vi "Volume ROI entry window.vi"(6 "# of planes":i32, 7 "Do not initialise selector values":bool, 8 "ZplaneIndex (zero based)":i32, 10 "Zoom (in)":dbl=1.0 min=1.0 max=10.0 step=0.10000000149011612, 11 "Coordinates":i32[](array[numeric])) -> (1 "Zoom (out)":dbl=1.0 min=1.0 max=10.0 step=0.10000000149011612, 3 "ROIs Info []":T1[](array[typedef]) {"Zoom" min=1.0 max=10.0 step=0.10000000149011612}, 4 "Cancelled":bool)   [LabVIEW 2013]
uses:
  Typedefs/ROI spec.ctl
  Typedefs/ROI ID Enum.ctl
  ROI Entry screen/Typedefs/Volume entry ctrl refs cluster.ctl
  <vilib>/Utility/miscctls.llb/LVPointTypeDef.ctl
  ROI Entry screen/Globals/gl_Volume Entry UI globals.vi
  ROI Entry screen/Globals/gl_ROI Entry UI globals.vi
panel:
  in  "Z-step (planes)":i32=1 min=1 max=17 step=1
  in  "Dual Rectangle":bool
  in  "Zoom":dbl=1.0 min=0.001 max=10.0 step=0.10000000149011612
  in  "Cancel":bool
  in  "Proceed":bool
  in  "Z-plane 2":u16(ring) caption="Z-plane" items=["Z-plane 1", "Z-plane 2", "Z-plane 3", "Z-plane 4", "Z-plane 5", "Z-plane 6", "Z-plane 7", "Z-plane 8", "Z-plane 9", "Z-plane 10", "Z-plane 11", "Z-plane 12", "Z-plane 13", "Z-plane 14", "Z-plane 15", "Z-plane 16", "Z-plane 17", "Z-plane 18", "Z-plane 19", "Z-plane 20", "Z-plane 21", "Z-plane 22", "Z-plane 23", "Z-plane 24", "Z-plane 25", "Z-plane 26", "Z-plane 27", "Z-plane 28", "Z-plane 29", "Z-plane 30", "Z-plane 31", "Z-plane 32", "Z-plane 33", "Z-plane 34", "Z-plane 35", "Z-plane 36", "Z-plane 37", "Z-plane 38", "Z-plane 39", "Z-plane 40", "Z-plane 41", "Z-plane 42", "Z-plane 43", "Z-plane 44", "Z-plane 45", "Z-plane 46", "Z-plane 47", "Z-plane 48", "Z-plane 49", "Z-plane 50", "Z-plane 51"]
  in  "Z-plane 1":u16(ring) caption="Z-plane" items=["Z-plane 1", "Z-plane 2", "Z-plane 3", "Z-plane 4", "Z-plane 5", "Z-plane 6", "Z-plane 7", "Z-plane 8", "Z-plane 9", "Z-plane 10", "Z-plane 11", "Z-plane 12", "Z-plane 13", "Z-plane 14", "Z-plane 15", "Z-plane 16", "Z-plane 17", "Z-plane 18", "Z-plane 19", "Z-plane 20", "Z-plane 21", "Z-plane 22", "Z-plane 23", "Z-plane 24", "Z-plane 25", "Z-plane 26", "Z-plane 27", "Z-plane 28", "Z-plane 29", "Z-plane 30", "Z-plane 31", "Z-plane 32", "Z-plane 33", "Z-plane 34", "Z-plane 35", "Z-plane 36", "Z-plane 37", "Z-plane 38", "Z-plane 39", "Z-plane 40", "Z-plane 41", "Z-plane 42", "Z-plane 43", "Z-plane 44", "Z-plane 45", "Z-plane 46", "Z-plane 47", "Z-plane 48", "Z-plane 49", "Z-plane 50", "Z-plane 51"]
  in  "Volume":bool
  # "To specify a volume from the drawn rectangle, tick the Volume box and select the z-planes between which the volume should be generated.\n \nTo draw two rectangles at precisely the same XY position but on different z-levels, tick the \"Dual Rectangle\" box."
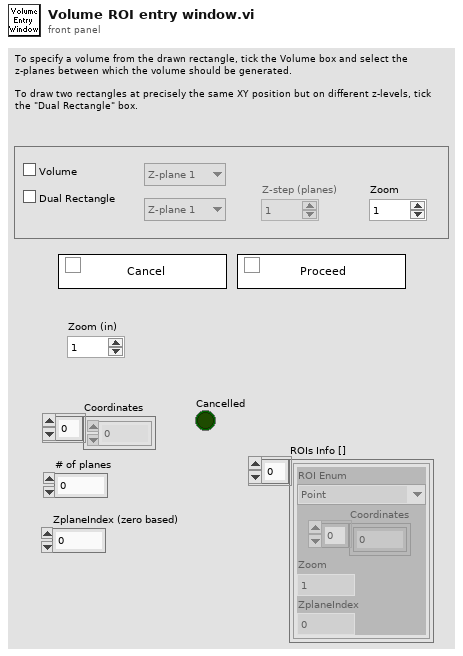
[diagram p1: front panel]
types:
  T1 = typedef "ROI spec.ctl" = cluster{"Coordinates":i32[], "Zoom":dbl, "ROI Enum":T2, "ZplaneIndex":i32}
  T2 = typedef "ROI ID Enum.ctl" = enum16{"Point", "MiniScan", "Comp. MiniScan", "Rectangle", "Comp. volume", "Arb. plane point"}
  T3 = typedef "Volume entry ctrl refs cluster.ctl" = cluster{"Z-step (planes)":refnum<vi>, "Volume":refnum<vi>, "Dual Rectangle":refnum<vi>, "Zoom":refnum<vi>, "Z-plane 1":refnum<vi>, "Z-plane 2":refnum<vi>, "ZplaneIndex (zero based)":refnum<vi>}
  T4 = typedef "LVPointTypeDef.ctl" = cluster{"Horizontal":i16, "Vertical":i16}
  T5 = enum8{"Enabled", "Disabled", "Disabled and Grayed Out"}
  T6 = typedef "ROI input mode.ctl" = enum16{"Unspecified", "Point-Line-Plane", "Volume"}
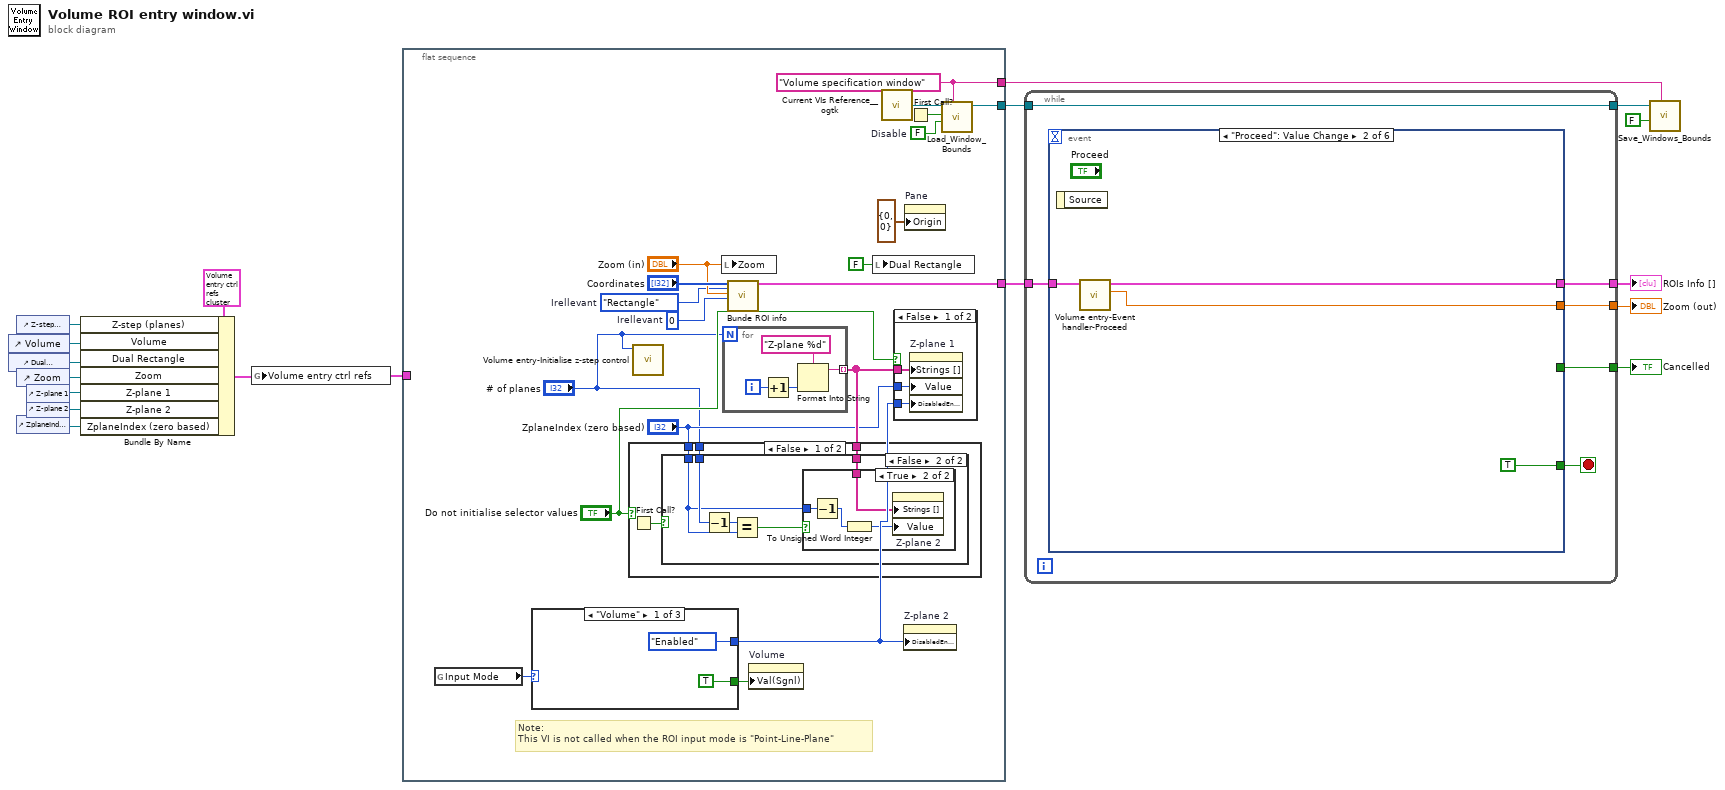
[diagram p0: block diagram]
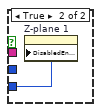
[diagram p2: hidden frame]
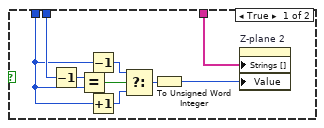
[diagram p3: hidden frame]
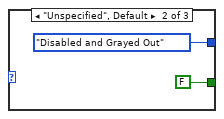
[diagram p6: hidden frame]
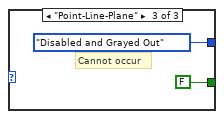
[diagram p7: hidden frame]
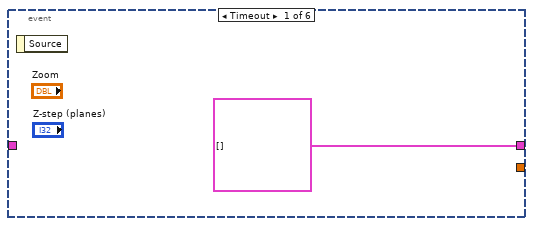
[diagram p8: hidden frame]
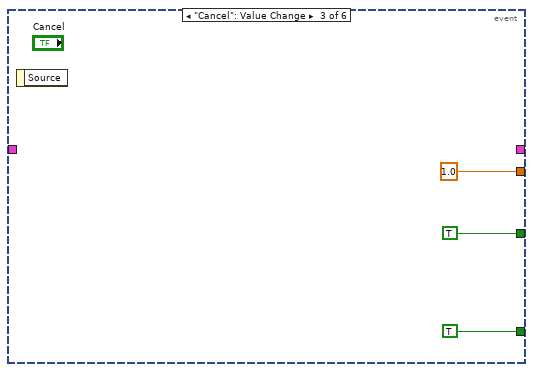
[diagram p9: hidden frame]
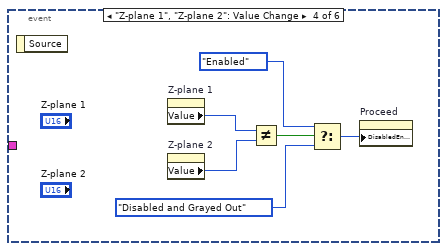
[diagram p10: hidden frame]
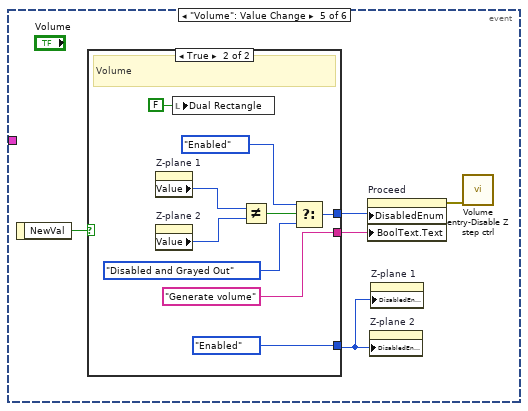
[diagram p11: hidden frame]
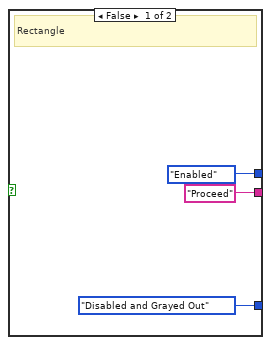
[diagram p12: hidden frame]
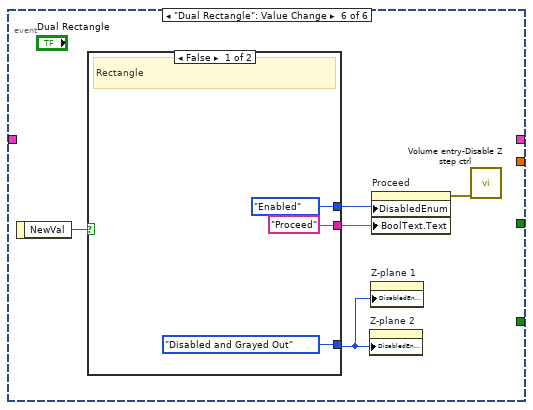
[diagram p13: hidden frame]
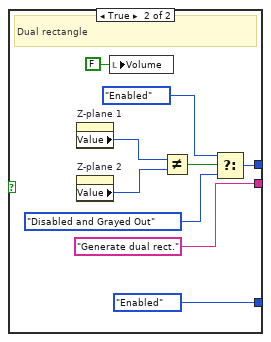
[diagram p14: hidden frame]
diagram:
  n1 = control-ref of="Volume"() -> (w6:refnum<vi>)
  n2 = control-ref of="Dual Rectangle"() -> (w5:refnum<vi>)
  n3 = control-ref of="Z-step (planes)"() -> (w8:refnum<vi>)
  n4 = control-ref of="Zoom"() -> (w4:refnum<vi>)
  n5 = control-ref of="ZplaneIndex (zero based)"() -> (w1:refnum<vi>)
  n6 = control-ref of="Z-plane 1"() -> (w3:refnum<vi>)
  n7 = control-ref of="Z-plane 2"() -> (w2:refnum<vi>)
  n8 = Bundle By Name(cluster=T3 {"Z-step (planes)"=refnum, "Volume"=refnum, "Dual Rectangle"=refnum, "Zoom"=refnum, "Z-plane 1"=refnum, "Z-plane 2"=refnum, "ZplaneIndex (zero based)"=refnum} ("Volume entry ctrl refs"), "Z-step (planes)"=w8, "Volume"=w6, "Dual Rectangle"=w5, "Zoom"=w4, "Z-plane 1"=w3, "Z-plane 2"=w2, "ZplaneIndex (zero based)"=w1) -> (w7:T3)
  n9 = global write "gl_Volume Entry UI globals.vi" "Volume entry ctrl refs"(w7) -> ()
  n10 = flat-sequence {
    tunnel: [w29] -> w15
    tunnel: [w25] -> w13
    tunnel: [w24] -> w11
    tunnel: w7 -> [_]
    frame #0 {
      w22 = 0  # Irellevant
      w23 = ROI_ID_Enum."Rectangle"  # Irellevant
      w26 = FALSE  # Disable
      w25 = "Volume specification window" ("Window Name (i.e. Key)")
      # "Note:\nThis VI is not called when the ROI input mode is \"Point-Line-Plane\""
      n11 = global read "gl_ROI Entry UI globals.vi" "Input Mode"() -> (w34:T6)
      n12 = case shown="\"Volume\"" w34 {
        tunnel: [TRUE ("Create Volume") FALSE ("Create Volume") FALSE ("Create Volume")] -> w33
        tunnel: [T5."Enabled" ("Disabled") T5."Disabled and Grayed Out" ("Disabled") T5."Disabled and Grayed Out" ("Disabled")] -> w19
        frame "Volume" {
        }
        frame "Unspecified", Default {
        }
        frame "Point-Line-Plane" {
          # "Cannot occur"
        }
      }
      n13 = call "Volume entry-Initialise z-step control.vi"("# of planes"="# of planes") -> ()  [unwired: 10 in, 1 out]
      n14 = local write "Zoom"("Zoom (in)") -> ()
      n15 = for {
        N: "# of planes" -> [_]
        tunnel: [w70] -> w36 mode=indexing
        i -> [w72]
        n16 = Increment(x=w72) -> (x+1=w71:i32)
        n17 = Format Into String(format string="Z-plane %d", w71) -> (resulting string=w70:string)  [unwired: 2 in, 1 out]
      }
      n18 = case shown="False" "Do not initialise selector values" {
        tunnel: w36 -> [w44 _]
        tunnel: "# of planes" -> [w43 _]
        tunnel: "ZplaneIndex (zero based)" -> [w42 _]
        frame False {
          n19 = First Call?() -> (First Call?: T/F=w41:bool)
          n20 = case shown="False" w41 {
            tunnel: w44 -> [w53 w58]
            tunnel: w43 -> [w52 w57]
            tunnel: w42 -> [w45 w55]
            frame True {
              n21 = Decrement(x=w52) -> (x-1=w51:i32)
              n22 = Equal?(x=w51, y=w45) -> (x = y?=w50:bool)
              n23 = Decrement(x=w45) -> (x-1=w48:i32)
              n24 = Increment(x=w45) -> (x+1=w49:i32)
              n25 = Select(t=w48, s=w50, f=w49) -> (s? t:f=w47:i32)
              n26 = To Unsigned Word Integer(number=w47) -> (unsigned 16bit integer=w46:u16)
              n27 = property on="Z-plane 2" class="Ring (strict)"("Strings []"=w53, "Value"=w46) -> ()  [unwired: 2 in, 2 out]
            }
            frame False {
              n28 = Decrement(x=w57) -> (x-1=w56:i32)
              n29 = Equal?(x=w56, y=w55) -> (x = y?=w54:bool)
              n30 = case shown="True" w54 {
                tunnel: w58 -> [_ w62]
                tunnel: w55 -> [_ w60]
                frame False {
                }
                frame True {
                  n31 = Decrement(x=w60) -> (x-1=w59:i32)
                  n32 = To Unsigned Word Integer(number=w59) -> (unsigned 16bit integer=w61:u16)
                  n33 = property on="Z-plane 2" class="Ring (strict)"("Strings []"=w62, "Value"=w61) -> ()  [unwired: 2 in, 2 out]
                }
              }
            }
          }
        }
        frame True {
        }
      }
      n34 = call "Bunde ROI info.vi"("ROI Coordinates"="Coordinates", "ROI Enum"=w23, "Zoom"="Zoom (in)", "ZplaneIndex"=w22) -> ("ROI Info"=w29:T1)  [unwired: 15 in]
      n35 = property on="Volume" class="Bool (strict)"("Val(Sgnl)"=w33) -> ()  [unwired: 2 in, 2 out]
      n36 = local write "Dual Rectangle"(FALSE ("Dual Rectangle")) -> ()
      n37 = call "Current VIs Reference__ogtk.vi"() -> ("Current VI's reference"=w28:refnum<vi>)  [unwired: 5 in]
      n38 = case shown="False" "Do not initialise selector values" {
        tunnel: w36 -> [w39 _]
        tunnel: "ZplaneIndex (zero based)" -> [w38 _]
        tunnel: w19 -> [w37 w40]
        frame False {
          n39 = property on="Z-plane 1" class="Ring (strict)"("Strings []"=w39, "Value"=w38, "DisabledEnum"=w37) -> ()  [unwired: 2 in, 2 out]
        }
        frame True {
          n40 = property on="Z-plane 1" class="Ring (strict)"("DisabledEnum"=w40) -> ()  [unwired: 2 in, 2 out]
        }
      }
      n41 = property on="Z-plane 2" class="Ring (strict)"("DisabledEnum"=w19) -> ()  [unwired: 2 in, 2 out]
      n42 = property on="Pane" class="Pane"("Origin"=T4 {"Horizontal"=0, "Vertical"=0}) -> ()  [unwired: 2 in, 2 out]
      n43 = First Call?() -> (First Call?: T/F=w27:bool)
      n44 = call "Load_Window_Bounds.vi"("Window Name (i.e. Key)"=w25, "Disable"=w26, "First Call"=w27, "Window VI's Ref"=w28) -> ("reference out"=w24:refnum<vi>)  [unwired: 4 in, 3 out]
    }
  }
  n45 = while {
    tunnel: [w78] -> w17
    tunnel: w15 -> [w77]
    tunnel: [w75] -> w16
    tunnel: [w74] -> w14
    tunnel: w11 -> [w73]
    tunnel: [w73] -> w10
    stop <- w76 stop-if-true
    n46 = event shown="[1] \"Proceed\": Value Change" {
      selector: _ -> [_ _ _ _ _ _]
      dyn-events: _ -> [_ _ _ _ _ _]
      timeout: _ -> [_ _ _ _ _ _]
      tunnel: [T1[] [] ("ROIs Info []") w83 _ _ _ _] -> w78
      tunnel: w77 -> [_ w81 _ _ _ _]
      tunnel: [_ TRUE TRUE _ _ _] -> w76
      tunnel: [_ _ TRUE ("Cancel") _ _ _] -> w75
      tunnel: [_ w80 1.0 ("Zoom") _ _ _] -> w74
      event Timeout {
        n47 = event-data() -> ()  [unwired: 1 in, 1 out]
      }
      event "Proceed": Value Change {
        n48 = event-data() -> ()  [unwired: 1 in, 1 out]
        n49 = call "Volume entry-Event handler-Proceed.vi"("ROI Info"=w81) -> ("Zoom"=w80:dbl, "ROI Info []"=w83:T1[])  [unwired: 9 in]
      }
      event "Cancel": Value Change {
        n50 = event-data() -> ()  [unwired: 1 in, 1 out]
      }
      event "Z-plane 1", "Z-plane 2": Value Change {
        n51 = event-data() -> ()  [unwired: 1 in, 1 out]
        n52 = property on="Z-plane 1" class="Ring (strict)"() -> ("Value"=w92:u16)  [unwired: 2 in, 2 out]
        n53 = property on="Z-plane 2" class="Ring (strict)"() -> ("Value"=w91:u16)  [unwired: 2 in, 2 out]
        n54 = Not Equal?(x=w92, y=w91) -> (x != y?=w90:bool)
        n55 = Select(t=T5."Enabled" ("Disabled"), s=w90, f=T5."Disabled and Grayed Out" ("Disabled")) -> (s? t:f=w87:T5)
        n56 = property on="Proceed" class="Bool"("DisabledEnum"=w87) -> ()  [unwired: 2 in, 2 out]
      }
      event "Volume": Value Change {
        n57 = event-data() -> ("NewVal"=w96:bool)  [unwired: 1 in]
        n58 = case shown="True" w96 {
          tunnel: [T5."Enabled" ("Disabled") w104] -> w97
          tunnel: [T5."Disabled and Grayed Out" ("Disabled") T5."Enabled" ("Disabled")] -> w95
          tunnel: ["Proceed" "Generate volume"] -> w94
          frame False {
            # "Rectangle"
          }
          frame True {
            # "Volume"
            n59 = property on="Z-plane 1" class="Ring (strict)"() -> ("Value"=w109:u16)  [unwired: 2 in, 2 out]
            n60 = property on="Z-plane 2" class="Ring (strict)"() -> ("Value"=w108:u16)  [unwired: 2 in, 2 out]
            n61 = local write "Dual Rectangle"(FALSE ("Dual Rectangle")) -> ()
            n62 = Not Equal?(x=w109, y=w108) -> (x != y?=w107:bool)
            n63 = Select(t=T5."Enabled" ("Disabled"), s=w107, f=T5."Disabled and Grayed Out" ("Disabled")) -> (s? t:f=w104:T5)
          }
        }
        n64 = property on="Proceed" class="Bool"("DisabledEnum"=w97, "BoolText.Text"=w94) -> (error out=w93:errorcluster)  [unwired: 2 in, 1 out]
        n65 = property on="Z-plane 2" class="Ring (strict)"("DisabledEnum"=w95) -> ()  [unwired: 2 in, 2 out]
        n66 = property on="Z-plane 1" class="Ring (strict)"("DisabledEnum"=w95) -> ()  [unwired: 2 in, 2 out]
        n67 = call "Volume entry-Disable Z step ctrl.vi"("error in (no error)"=w93) -> ()  [unwired: 10 in, 1 out]
      }
      event "Dual Rectangle": Value Change {
        n68 = event-data() -> ("NewVal"=w112:bool)  [unwired: 1 in]
        n69 = case shown="False" w112 {
          tunnel: [T5."Enabled" ("Disabled") w121] -> w114
          tunnel: [T5."Disabled and Grayed Out" ("Disabled") T5."Enabled" ("Disabled")] -> w113
          tunnel: ["Proceed" "Generate dual rect."] -> w111
          frame False {
            # "Rectangle"
          }
          frame True {
            # "Dual rectangle"
            n70 = property on="Z-plane 1" class="Ring (strict)"() -> ("Value"=w126:u16)  [unwired: 2 in, 2 out]
            n71 = property on="Z-plane 2" class="Ring (strict)"() -> ("Value"=w125:u16)  [unwired: 2 in, 2 out]
            n72 = local write "Volume"(FALSE ("Volume")) -> ()
            n73 = Not Equal?(x=w126, y=w125) -> (x != y?=w124:bool)
            n74 = Select(t=T5."Enabled" ("Disabled"), s=w124, f=T5."Disabled and Grayed Out" ("Disabled")) -> (s? t:f=w121:T5)
          }
        }
        n75 = property on="Z-plane 2" class="Ring (strict)"("DisabledEnum"=w113) -> ()  [unwired: 2 in, 2 out]
        n76 = property on="Z-plane 1" class="Ring (strict)"("DisabledEnum"=w113) -> ()  [unwired: 2 in, 2 out]
        n77 = property on="Proceed" class="Bool"("DisabledEnum"=w114, "BoolText.Text"=w111) -> (error out=w110:errorcluster)  [unwired: 2 in, 1 out]
        n78 = call "Volume entry-Disable Z step ctrl.vi"("error in (no error)"=w110) -> ()  [unwired: 10 in, 1 out]
      }
    }
  }
  "ROIs Info []" <- w17
  "Cancelled" <- w16
  "Zoom (out)" <- w14
  n79 = call "Save_Windows_Bounds.vi"("Window Name (i.e. Key)"=w13, "Front Panel Window:Open"=FALSE, "Window VI's Ref"=w10) -> ()  [unwired: 8 in, 1 out]
